vi "HexStr2Int.vi"(10 "十六进制字符串":string) -> (1 "数字":u32)   [LabVIEW 2017]
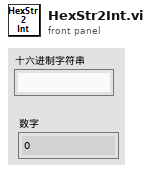
[diagram p1: front panel]
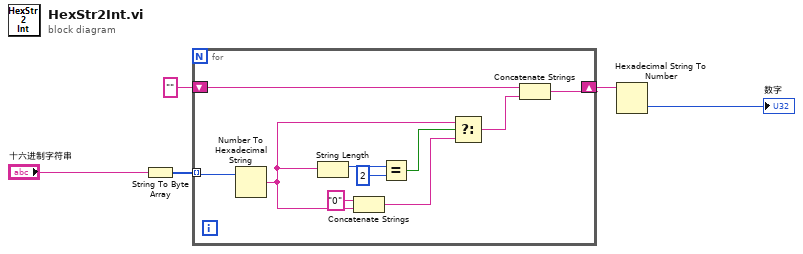
[diagram p0: block diagram]
diagram:
  n1 = String To Byte Array(string="十六进制字符串") -> (unsigned byte array=w3:u8[])
  n2 = for {
    shift-right: [w6] -> w2
    shift-left: "" -> [w8]
    tunnel: w3 -> [w15] mode=indexing
    n3 = Number To Hexadecimal String(2:w15) -> (0:w11:string)  [unwired: 1 in]
    n4 = String Length(string=w11) -> (length=w14:i32)
    n5 = Concatenate Strings("0" ("字符串"), w11) -> (w9:string)
    n6 = Equal?(x=w14, y=2) -> (x = y?=w12:bool)
    n7 = Select(t=w11, s=w12, f=w9) -> (s? t:f=w7:string)
    n8 = Concatenate Strings(w8, w7) -> (w6:string)
  }
  n9 = Hexadecimal String To Number(string=w2) -> (number=→"数字":u32)  [unwired: 2 in, 1 out]
